vi "Presynthesize.vi"(0 "Channel in":refnum<class "Channel.lvclass">, 5 "Fs (Hz)":dbl, 7 "Npts":i32, 9 "Repetition":i32, 11 "error in (no error)":errorcluster) -> (4 "Channel out":refnum<class "Channel.lvclass">, 15 "error out":errorcluster)   [LabVIEW 2015, in "Channel.lvclass"]
uses:
  Channel.lvclass
  Channel.lvclass/Channel.ctl
  Waveforms/Waveform/Waveform.lvclass
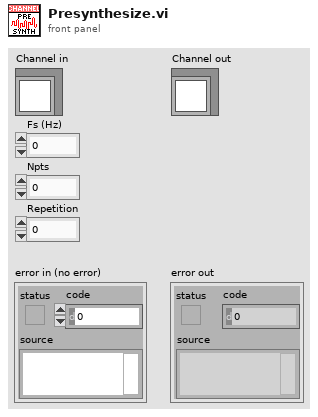
[diagram p1: front panel]
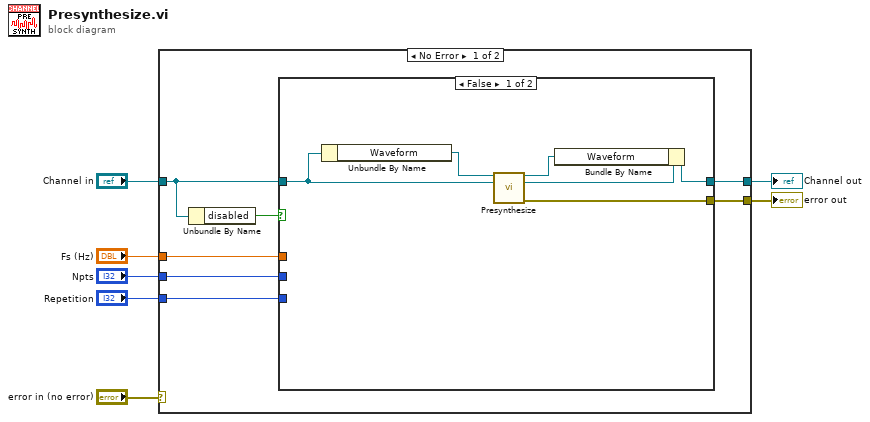
[diagram p0: block diagram]
diagram:
  n1 = case shown="No Error" "error in (no error)" {
    selector: "error in (no error)" -> [_ w23]
    tunnel: [w8 w23] -> w6
    tunnel: [w11 w22] -> w4
    tunnel: "Channel in" -> [w10 w22]
    tunnel: "Fs (Hz)" -> [w14 _]
    tunnel: "Npts" -> [w13 _]
    tunnel: "Repetition" -> [w12 _]
    frame No Error {
      n2 = Unbundle By Name(w10) -> ("disabled"=w9:bool)
      n3 = case shown="False" w9 {
        tunnel: w14 -> [_ _]
        tunnel: w13 -> [_ _]
        tunnel: w12 -> [_ _]
        tunnel: [w20 w21] -> w11
        tunnel: w10 -> [w18 w21]
        tunnel: [w15 _] -> w8
        frame False {
          n4 = Unbundle By Name(w18) -> ("Waveform"=w19:refnum<class "Waveform.lvclass">)
          n5 = call-dynamic "Presynthesize.vi"("Waveform in"=w19, "Channel in"=w18) -> ("Waveform out"=w16:refnum<class "Waveform.lvclass">, "Channel out"=w17:refnum<class "Channel.lvclass">, "error out"=w15:errorcluster)  [unwired: 11 in]
          n6 = Bundle By Name(cluster=w17, "Waveform"=w16) -> (w20:refnum<class "Channel.lvclass">)
        }
        frame True {
        }
      }
    }
    frame Error {
    }
  }
  "error out" <- w6
  "Channel out" <- w4
